vi "Init FPGA.vi"(8 "error in":errorcluster) -> (0 "error out":errorcluster, 2 "Chassis3FPGA":T1, 3 "Chassis1FPGA":T2)   [LabVIEW 2018]
uses:
  FPGA/FPGA VI Reference.ctl
  FPGA/Chassis3FPGARef.ctl
  <vilib>/FPGAPlugInAG/cRIO-9082/niLvFpga_Open_cRIO-9082.vi
  <vilib>/rvi/interface/common/dynamic/niFpgaDynamicAddResources.vi
  <vilib>/FPGAPlugInAG/Dynamic/niLvFpga_Run_Dynamic.vi
  <vilib>/FPGAPlugInAG/NI 9148/niLvFpga_Open_NI 9148.vi
  <vilib>/FPGAPlugInAG/Dynamic/niLvFpga_Reset_Dynamic.vi
  <vilib>/rvi/interface/nirviOpenFPGA/nirviOpenFPGA.xnode
  FPGA Bitfiles/APU_FPGA230220A.lvbitx
  <vilib>/rvi/interface/nirviMethod/nirviMethod.xnode
  FPGA Bitfiles/Chassis3FPGA20230223B.lvbitx
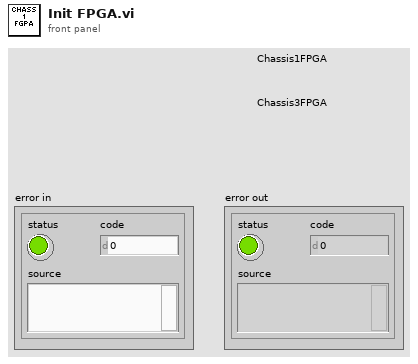
[diagram p1: front panel]
types:
  T1 = typedef "Chassis3FPGARef.ctl" = refnum<k20>
  T2 = typedef "FPGA VI Reference.ctl" = refnum<k20>
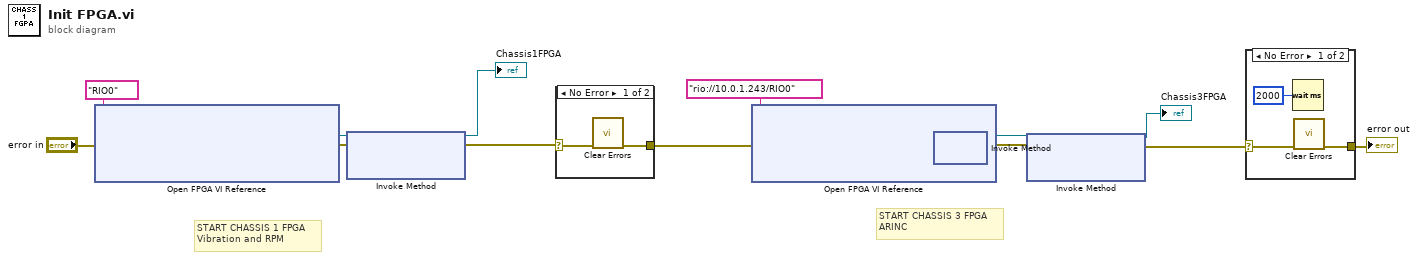
[diagram p0: block diagram]
diagram:
  # "START CHASSIS 3 FPGA\nARINC"
  # "START CHASSIS 1 FPGA\nVibration and RPM"
  n1 = xnode "Open FPGA VI Reference"("error in"="error in", "resource name"=tag "RIO0") -> ("FPGA VI Reference Out"=w9:refnum<k20>, "error out"=w10:errorcluster)
  n2 = xnode "Invoke Method"("FPGA VI Reference In"=w9, "error in"=w10) -> ("FPGA VI Reference Out"=→"Chassis1FPGA":refnum<k20>, "error out"=w2:errorcluster)  [unwired: 1 in]
  n3 = case shown="No Error" w2 {
    selector: w2 -> [w17 w18]
    tunnel: [w16 w18] -> w1
    frame No Error {
      n4 = call <vilib>:"Clear Errors.vi"("error in (no error)"=w17) -> ("error out"=w16:errorcluster)  [unwired: 5 in, 1 out]
    }
    frame Error {
    }
  }
  n5 = xnode "Open FPGA VI Reference"("error in"=w1, "resource name"=tag "rio://10.0.1.243/RIO0") -> ("FPGA VI Reference Out"=w8:refnum<k20>, "error out"=w7:errorcluster)
  n6 = xnode "Invoke Method"("FPGA VI Reference In"=w8, "error in"=w7) -> ("FPGA VI Reference Out"=w6:refnum<k20>, "error out"=w5:errorcluster)
  n7 = xnode "Invoke Method"("FPGA VI Reference In"=w6, "error in"=w5) -> ("FPGA VI Reference Out"=→"Chassis3FPGA":refnum<k20>, "error out"=w3:errorcluster)  [unwired: 1 in]
  n8 = case shown="No Error" w3 {
    selector: w3 -> [w21 w22]
    tunnel: [w19 w22] -> w15
    frame No Error {
      n9 = Wait (ms)(milliseconds to wait=u32 2000) -> ()  [unwired: 1 out]
      n10 = call <vilib>:"Clear Errors.vi"("error in (no error)"=w21) -> ("error out"=w19:errorcluster)  [unwired: 5 in, 1 out]
    }
    frame Error {
    }
  }
  "error out" <- w15
